vi "EnumControlToJson.vi"(8 "error in (no error)":errorcluster, 10 "Owner Bounds":T1, 11 "NamedNumeric in":refnum<vi>) -> (0 "error out":errorcluster, 3 "String":string)   [LabVIEW 2017]
uses:
  <vilib>/Utility/miscctls.llb/LVRectTypeDef.ctl
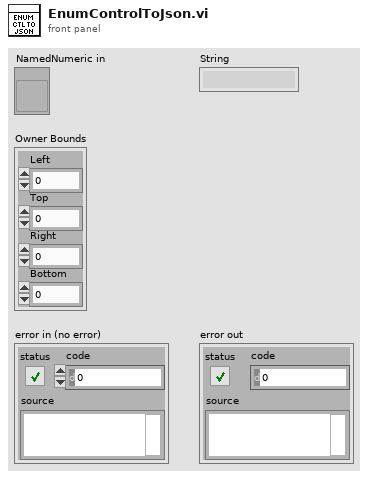
[diagram p1: front panel]
types:
  T1 = typedef "LVRectTypeDef.ctl" = cluster{"Left":i16, "Top":i16, "Right":i16, "Bottom":i16}
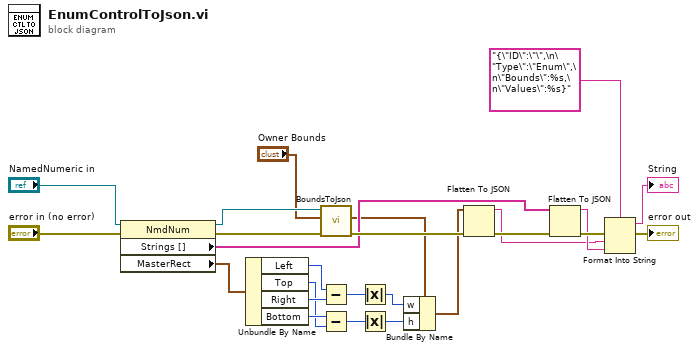
[diagram p0: block diagram]
diagram:
  n1 = property class="NmdNum"(reference="NamedNumeric in", error in="error in (no error)") -> (reference out=w18:refnum<vi>, error out=w19:errorcluster, "Strings []"=w14:string[], "MasterRect"=w10:T1)
  n2 = Unbundle By Name(w10) -> ("Left"=w8:i16, "Top"=w5:i16, "Right"=w9:i16, "Bottom"=w6:i16)
  n3 = call "BoundsToJson.vi"("error in (no error)"=w19, "Owner Bounds"="Owner Bounds", "GObj in"=w18) -> ("error out"=w20:errorcluster, "Relative Bounds"=w12:cluster{"x":i32, "y":i32, "w":i32, "h":i32})  [unwired: 5 in, 2 out]
  n4 = Subtract(x=w8, y=w9) -> (x-y=w7:i16)
  n5 = Subtract(x=w6, y=w5) -> (x-y=w4:i16)
  n6 = Absolute Value(x=w7) -> (abs(x)=w3:i16)
  n7 = Absolute Value(x=w4) -> (abs(x)=w2:i16)
  n8 = Bundle By Name(cluster=w12, "w"=w3, "h"=w2) -> (w11:cluster{"x":i32, "y":i32, "w":i32, "h":i32})
  n9 = Flatten To JSON(anything=w11, error in (no error)=w20) -> (JSON string=w1:string, 11:w21:errorcluster)  [unwired: 1 in]
  n10 = Flatten To JSON(anything=w14, error in (no error)=w21) -> (JSON string=w13:string, 11:w22:errorcluster)  [unwired: 1 in]
  n11 = Format Into String(format string="{\"ID\":\"\",\n\"Type\":\"Enum\",\n\"Bounds\":%s,\n\"Values\":%s}", error in=w22, w1, w13) -> (resulting string=→"String":string, error out=→"error out":errorcluster)  [unwired: 1 in]
